vi "Init WebView2 Core.vi"(8 "error in (no error)":errorcluster, 10 "Display State In":T1, 11 "WebView In":refnum<k24>) -> (0 "error out":errorcluster, 2 "Display State In 2":T1={"WebView2 Ref"=refnum, "event callback refnum"=refnum, "Events"={"Navigation Complete Event"=refnum, "Source Changed Event"=refnum, "Document Title Changed Event"=refnum, "Status Bar Text Changed"=refnum, "Web Message Received"=refnum, "Window Close Requested"=refnum, "DOM Loaded"=refnum}, "Paths"={"Webview2 Native"=path "C:/Users/kleins/Desktop/webview2/microsoft.web.webview2.1.0.1370.28/build/native", "Edge Application"=path "", "User Data"=path ""}, "Environment Options"={"additionalBrowserArguments"="", "language"="", "targetCompatibleBrowserVersion"="", "allowSingleSignOnUsingOSPrimaryAccount"=FALSE}}, 3 "CoreWebView Out":refnum<k24>)   [LabVIEW 2020, in "WebView2 Control.xctl"]
uses:
  WebView2 Control.xctl
  E:/Labview/LV 2020/Libs/WebView2/LV-WebView2/Source/Libs/Microsoft.Web.WebView2.Core.dll
  Libs/Microsoft.Web.WebView2.Core.dll
  State.ctl
  E:/Labview/LV 2020/Libs/WebView2/LV-WebView2/Source/Libs/Microsoft.Web.WebView2.WinForms.dll
  Libs/Microsoft.Web.WebView2.WinForms.dll
  Events.ctl
  Paths.ctl
  Core Env Options.ctl
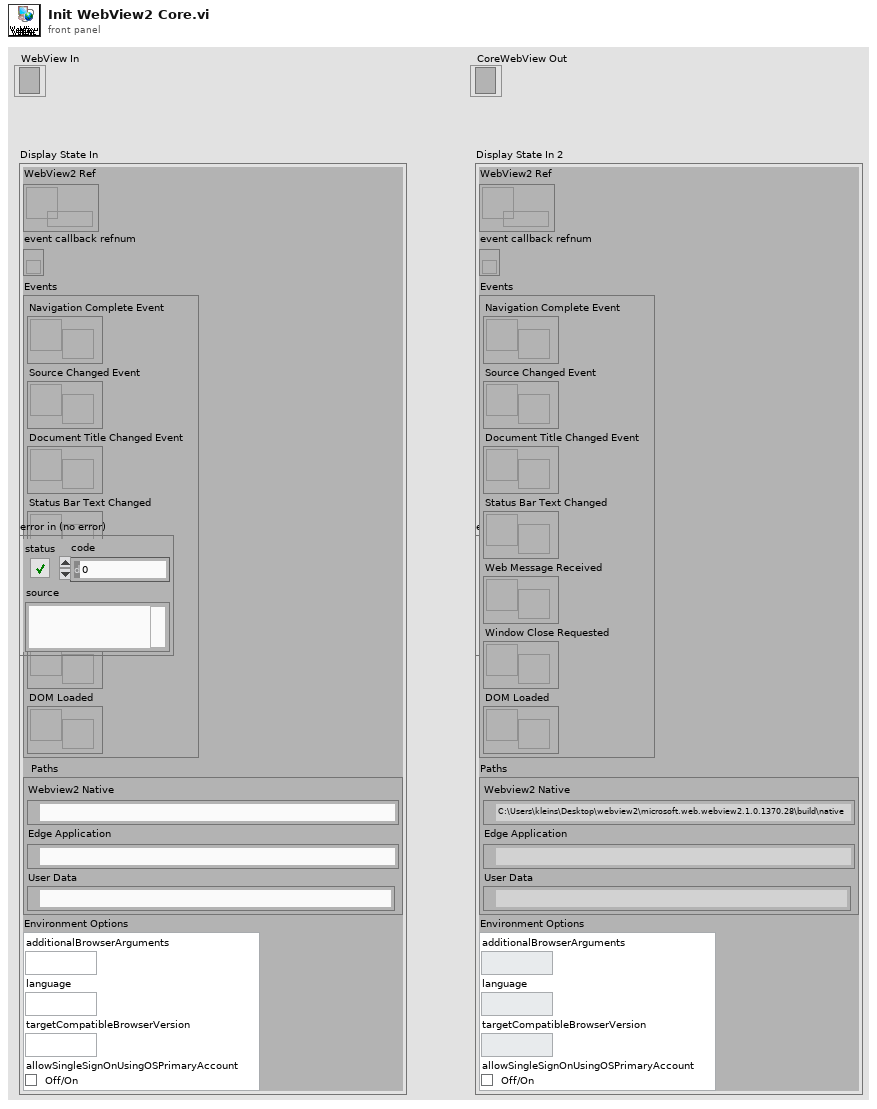
[diagram p1: front panel]
types:
  T1 = typedef "WebView2 Control.xctl/State.ctl" = cluster{"WebView2 Ref":refnum<data-value>, "event callback refnum":refnum<k27>, "Events":T2, "Paths":T3, "Environment Options":T4}
  T2 = typedef "WebView2 Control.xctl/Events.ctl" = cluster{"Navigation Complete Event":refnum<user-event>, "Source Changed Event":refnum<user-event>, "Document Title Changed Event":refnum<user-event>, "Status Bar Text Changed":refnum<user-event>, "Web Message Received":refnum<user-event>, "Window Close Requested":refnum<user-event>, "DOM Loaded":refnum<user-event>}
  T3 = typedef "WebView2 Control.xctl/Paths.ctl" = cluster{"Webview2 Native":path, "Edge Application":path, "User Data":path}
  T4 = typedef "WebView2 Control.xctl/Core Env Options.ctl" = cluster{"additionalBrowserArguments":string, "language":string, "targetCompatibleBrowserVersion":string, "allowSingleSignOnUsingOSPrimaryAccount":bool}
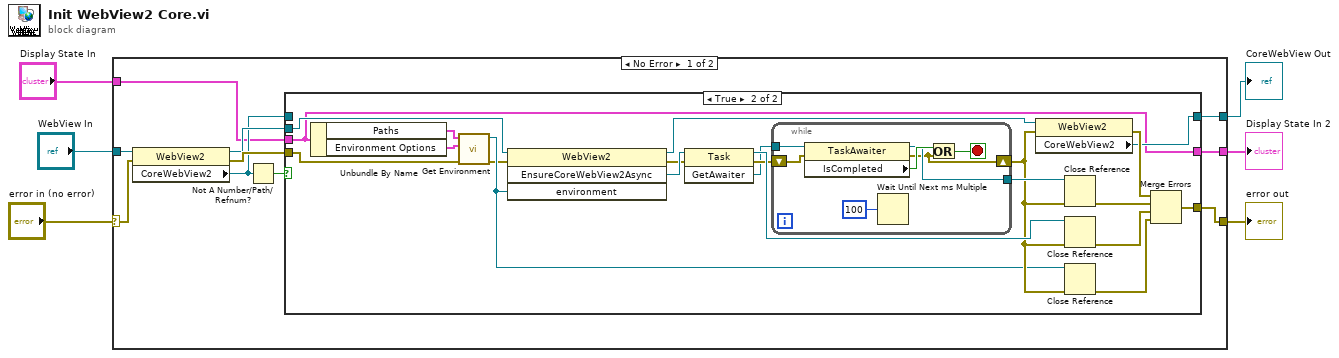
[diagram p0: block diagram]
diagram:
  n1 = case shown="No Error" "error in (no error)" {
    selector: "error in (no error)" -> [w9 w49]
    tunnel: [w16 _] -> w6
    tunnel: [w14 w49] -> w5
    tunnel: "WebView In" -> [w10 _]
    tunnel: [w8 w48] -> w2
    tunnel: "Display State In" -> [w7 w48]
    frame No Error {
      n2 = property class="WebView2"(reference=w10, error in=w9) -> (reference out=w13:refnum<k24>, error out=w15:errorcluster, "CoreWebView2"=w12:refnum<k24>)
      n3 = Not A Number/Path/Refnum?(number/path/refnum=w12) -> (NaN/Path/Refnum?=w11:bool)
      n4 = case shown="True" w11 {
        tunnel: [w19 w27] -> w16
        tunnel: w12 -> [w19 _]
        tunnel: w13 -> [_ w32]
        tunnel: w7 -> [w17 w26]
        tunnel: w15 -> [w18 w24]
        tunnel: [w18 w23] -> w14
        tunnel: [w17 w26] -> w8
        frame False {
        }
        frame True {
          n5 = Unbundle By Name(w26) -> ("Paths"=w25:T3, "Environment Options"=w20:T4)
          n6 = call "Get Environment.vi"("error in"=w24, 10:w20, "Paths"=w25) -> ("error out"=w21:errorcluster, "Environment out"=w22:refnum<k24>)  [unwired: 7 in]
          n7 = invoke class="WebView2" method="EnsureCoreWebView2Async"(reference=w32, error in=w21, "environment"=w22) -> (reference out=w39:refnum<k24>, error out=w37:errorcluster, "EnsureCoreWebView2Async"=w38:refnum<k24>)  [unwired: 1 in, 1 out]
          n8 = invoke class="Task" method="GetAwaiter"(reference=w38, error in=w37) -> (reference out=w36:refnum<k24>, error out=w31:errorcluster, "GetAwaiter"=w30:refnum<k24>)  [unwired: 1 in]
          n9 = while {
            tunnel: w30 -> [w46]
            shift-right: [w41] -> w28
            shift-left: w31 -> [w47]
            tunnel: [w43] -> w34
            stop <- w42 stop-if-true
            n10 = property class="TaskAwaiter"(reference=w46, error in=w47) -> (reference out=w43:refnum<k24>, error out=w41:errorcluster, "IsCompleted"=w44:bool)
            n11 = Wait Until Next ms Multiple(millisecond multiple=u32 100) -> ()  [unwired: 1 out]
            n12 = Or(x=w44, y=w41) -> (x .or. y?=w42:bool)
          }
          n13 = property class="WebView2"(reference=w39, error in=w28) -> (error out=w40:errorcluster, "CoreWebView2"=w27:refnum<k24>)  [unwired: 1 out]
          n14 = Close Reference(reference=w34, error in (no error)=w28) -> (error out=w33:errorcluster)
          n15 = Close Reference(reference=w36, error in (no error)=w28) -> (error out=w35:errorcluster)
          n16 = Close Reference(reference=w22, error in (no error)=w28) -> (error out=w29:errorcluster)
          n17 = Merge Errors(w40, w33, w35, w29) -> (w23:errorcluster)
        }
      }
    }
    frame Error {
    }
  }
  "CoreWebView Out" <- w6
  "error out" <- w5
  "Display State In 2" <- w2
